vi "GenerateCode.vi"(0 "XRef":T15, 1 "Terms":T12, 2 "Diagram":T11, 3 "State In":T1 {"BlockNodeState"."Draw Style" items=["FunctionBlock", "ExpressVI", "Variable", "Elemental I/O", "32x32 Icon", "FunctionBlockCompact"]; "BlockNodeState"."Terminal Data"."Terminal Flags" format="%.0b"}) -> (14 "Generated Code?":T10, 15 "Reply":T8, 16 "State Out":T1 {"BlockNodeState"."Draw Style" items=["FunctionBlock", "ExpressVI", "Variable", "Elemental I/O", "32x32 Icon", "FunctionBlockCompact"]; "BlockNodeState"."Terminal Data"."Terminal Flags" format="%.0b"})   [LabVIEW 2020, in "Set DDT Attributes.lvlib" / "Set DDT Properties.xnode"]
uses:
  <vilib>/express/express signal manip/GetorSetDDTAttributes/Set DDT Attributes/Set DDT Properties.xnode
  <vilib>/XNodeSupport/XNodeXNodeRef.ctl
  <vilib>/XNodeSupport/XNodeTermIDPairs.ctl
  <vilib>/XNodeSupport/XNodeTermIDPair.ctl
  <vilib>/XNodeSupport/XNodeTermRef.ctl
  <vilib>/XNodeSupport/XNodeString.ctl
  <vilib>/XNodeSupport/XNodeTopLevelDiagramRef.ctl
  <vilib>/express/express signal manip/GetorSetDDTAttributes/Set DDT Attributes/State.ctl
  <vilib>/BlockNodeSupport/BlockNodeState.ctl
  <vilib>/BlockNodeSupport/TerminalData.ctl
  <vilib>/picture/picture.llb/imagedata.ctl
  <vilib>/express/express signal manip/GetorSetDDTAttributes/Shared VIs/Attributes data.ctl
  <vilib>/express/express signal manip/GetorSetDDTAttributes/Shared VIs/Input.ctl
  <vilib>/express/express signal manip/GetorSetDDTAttributes/Shared VIs/Attributes name.ctl
  <vilib>/XNodeSupport/XNodeBool.ctl
  <vilib>/XNodeSupport/XNodeStringArray.ctl
  <vilib>/express/express signal manip/GetorSetDDTAttributes/Shared VIs/GetSetShared.lvlib
  <vilib>/XNodeSupport/NI_XNodeSupport.lvlib
  <vilib>/express/express signal manip/GetorSetDDTAttributes/Set DDT Attributes/Set DDT Attributes.lvlib
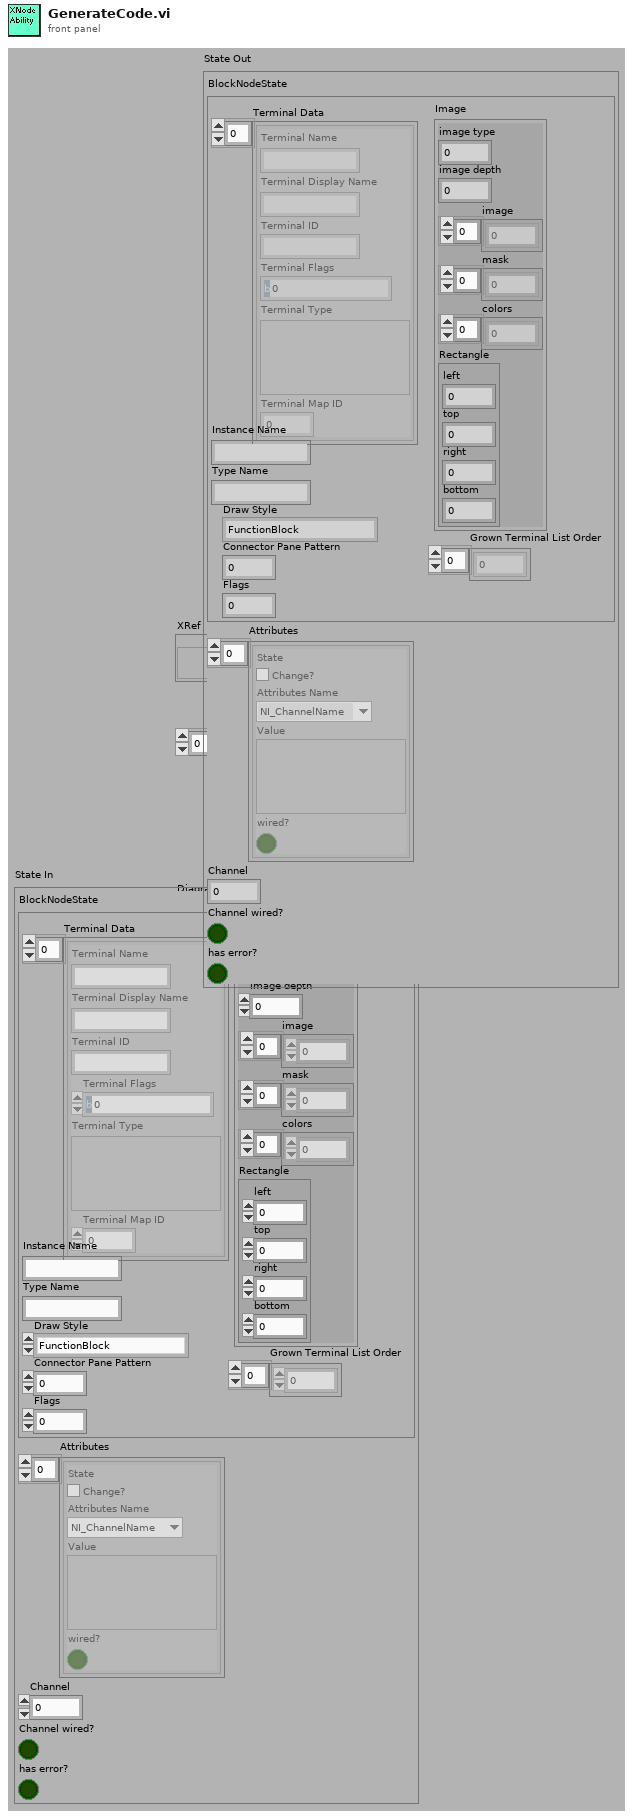
[diagram p1: front panel]
types:
  T1 = typedef "Set DDT Attributes.lvlib/Set DDT Properties.xnode/State.ctl" = cluster{"BlockNodeState":T2, "Attributes":T5[], "Channel":u32, "Channel wired?":bool, "has error?":bool}
  T2 = typedef "BlockNodeState.ctl" = cluster{"Terminal Data":T3[], "Instance Name":string, "Type Name":string, "Draw Style":i32, "Connector Pane Pattern":i32, "Flags":i32, "Grown Terminal List Order":i32[], "Image":T4}
  T3 = typedef "TerminalData.ctl" = cluster{"Terminal Name":string, "Terminal Display Name":string, "Terminal ID":string, "Terminal Flags":i32, "Terminal Type":variant, "Terminal Map ID":i32}
  T4 = typedef "imagedata.ctl" = cluster{"image type":i32, "image depth":i32, "image":u8[], "mask":u8[], "colors":u32[], "Rectangle":cluster{"left":i16, "top":i16, "right":i16, "bottom":i16}}
  T5 = typedef "GetSetShared.lvlib/Attributes data.ctl" = cluster{"State":T6, "Attributes Name":T7, "Value":variant, "wired?":bool}
  T6 = typedef "GetSetShared.lvlib/Input.ctl" = bool
  T7 = typedef "GetSetShared.lvlib/Attributes name.ctl" = enum16{"NI_ChannelName", "NI_ExpIsRelativeTime", "NI_ExpTimeStamp", "NI_ExpStartTimeStamp", "NI_ExpXDimension", "NI_UnitDescription"}
  T8 = typedef "NI_XNodeSupport.lvlib/XNodeStringArray.ctl" = T9[]
  T9 = typedef "NI_XNodeSupport.lvlib/XNodeString.ctl" = string
  T10 = typedef "NI_XNodeSupport.lvlib/XNodeBool.ctl" = bool
  T11 = typedef "NI_XNodeSupport.lvlib/XNodeTopLevelDiagramRef.ctl" = refnum<vi>
  T12 = typedef "NI_XNodeSupport.lvlib/XNodeTermIDPairs.ctl" = T13[]
  T13 = typedef "NI_XNodeSupport.lvlib/XNodeTermIDPair.ctl" = cluster{"Term":T14, "Id":T9}
  T14 = typedef "NI_XNodeSupport.lvlib/XNodeTermRef.ctl" = refnum<vi>
  T15 = typedef "NI_XNodeSupport.lvlib/XNodeXNodeRef.ctl" = refnum<vi>
  T16 = typedef "LVPointTypeDef.ctl" = cluster{"Horizontal":i16, "Vertical":i16}
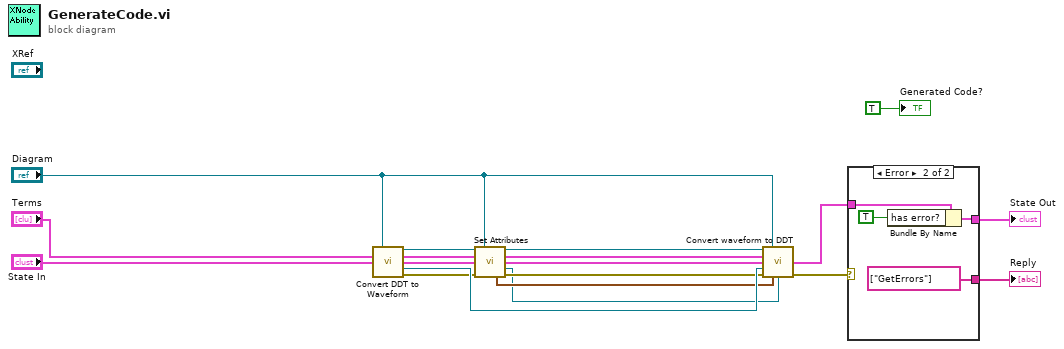
[diagram p0: block diagram]
diagram:
  n1 = call <vilib>:"Convert DDT to Waveform.vi"("Diagram"="Diagram", "Terms in"="Terms", "State In"="State In") -> ("Signal Ref out"=w16:refnum<vi>, "Terms out"=w17:T12, "State Out"=w13:T1, "Singals array ref"=w14:refnum<vi>, "error out"=w12:errorcluster)  [unwired: 2 in, 6 out]
  n2 = call <vilib>:"Set Attributes.vi"("Signal Ref in"=w16, "Diagram"="Diagram", "Terms"=w17, "State In"=w13, "error in"=w12) -> ("Signal Ref out"=w11:refnum<vi>, "Terms out"=w10:T12, "State Out"=w8:T1, "Error refence"=w5:T14, "Position"=w9:T16, "error out"=w7:errorcluster)  [unwired: 5 out]
  n3 = call <vilib>:"Convert waveform to DDT.vi"("modified Signal Ref"=w11, "Diagram"="Diagram", "Terms in"=w10, "State In"=w8, "Signals array Ref"=w14, "error in (no error)"=w7, "Position"=w9, "Error refence"=w5) -> ("State Out"=w2:T1, "error out"=w3:errorcluster)  [unwired: 6 out]
  n4 = case shown="Error" w3 {
    tunnel: [_ T8 ["GetErrors"] ("Reply")] -> w4
    tunnel: w2 -> [w20 w23]
    tunnel: [w20 w21] -> w1
    frame No Error {
    }
    frame Error {
      n5 = Bundle By Name(cluster=w23, "has error?"=TRUE) -> (w21:T1)
    }
  }
  "Reply" <- w4
  "State Out" <- w1
  "Generated Code?" <- T10 TRUE ("Generated Code?")
